vi "przeliczanie_kata.vi"(0 "24 bit":u8, 1 "16 bit":u8, 2 "8 bit":u8, 3 "najnizsze":u8) -> (7 "Numeric out":dbl)   [LabVIEW 2012]
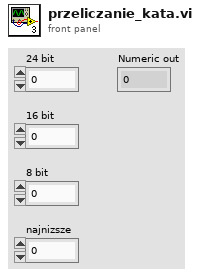
[diagram p1: front panel]
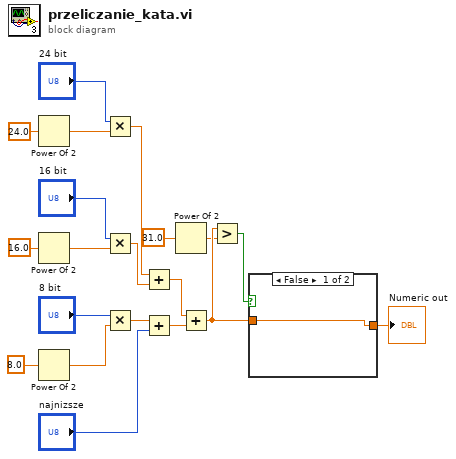
[diagram p0: block diagram]
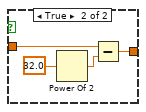
[diagram p2: hidden frame]
diagram:
  n1 = Power Of 2(x=24.0) -> (2^x=w2:dbl)
  n2 = Power Of 2(x=16.0) -> (2^x=w7:dbl)
  n3 = Power Of 2(x=8.0) -> (2^x=w6:dbl)
  n4 = Multiply(x="24 bit", y=w2) -> (x*y=w13:dbl)
  n5 = Multiply(x="16 bit", y=w7) -> (x*y=w12:dbl)
  n6 = Multiply(x="8 bit", y=w6) -> (x*y=w10:dbl)
  n7 = Add(x=w13, y=w12) -> (x+y=w15:dbl)
  n8 = Add(x=w10, y="najnizsze") -> (x+y=w14:dbl)
  n9 = Power Of 2(x=31.0) -> (2^x=w18:dbl)
  n10 = Add(x=w15, y=w14) -> (x+y=w19:dbl)
  n11 = Greater?(x=w19, y=w18) -> (0:w16:bool)
  n12 = case shown="False" w16 {
    tunnel: w19 -> [w21 w25]
    tunnel: [w21 w22] -> w20
    frame False {
    }
    frame True {
      n13 = Power Of 2(x=32.0) -> (2^x=w23:dbl)
      n14 = Subtract(x=w25, y=w23) -> (x-y=w22:dbl)
    }
  }
  "Numeric out" <- w20
